vi "TempAcqSubVI.vi"(8 "error in (no error)":errorcluster, 11 "Data Cluster in":T1) -> (0 "error out":errorcluster, 2 "Temperature":dbl, 3 "Data Cluster out":T1)   [LabVIEW 2017]
uses:
  Controls/ShiftRegisterCluster.ctl
  <vilib>/DAQmx/read.llb/DAQmx Read (Analog DBL 1Chan 1Samp).vi
  <vilib>/DAQmx/miscellaneous.llb/DAQmx Fill In Error Info.vi
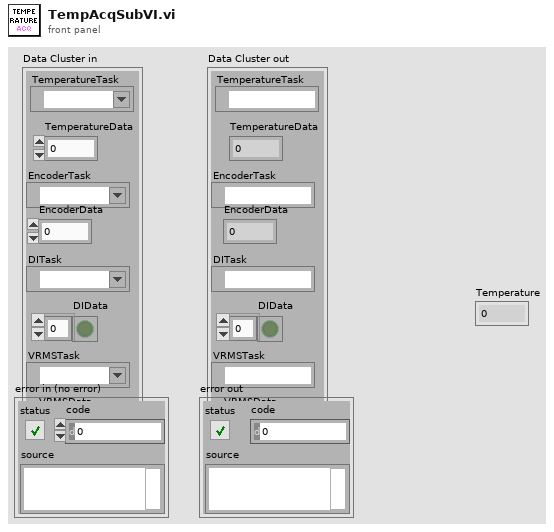
[diagram p1: front panel]
types:
  T1 = typedef "ShiftRegisterCluster.ctl" = cluster{"TemperatureTask":refnum<k21>, "TemperatureData":dbl, "EncoderTask":refnum<k21>, "EncoderData":dbl, "DITask":refnum<k21>, "DIData":bool[], "VRMSTask":refnum<k21>, "VRMSData":dbl, "FreqData":dbl}
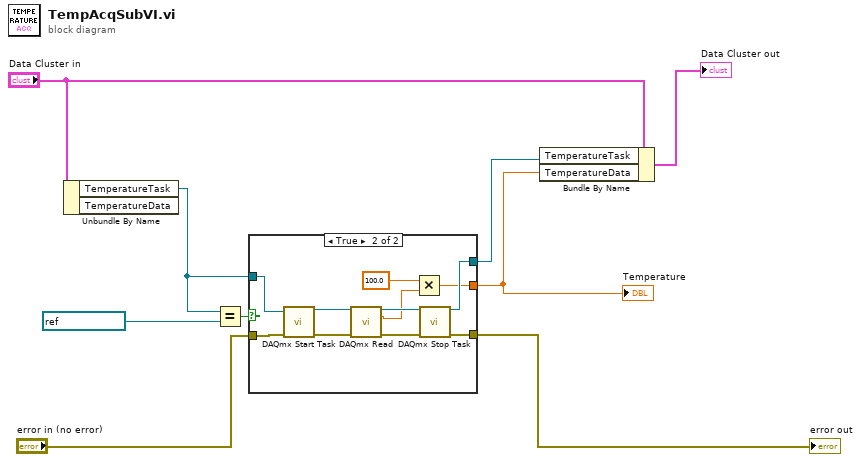
[diagram p0: block diagram]
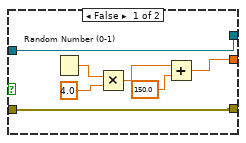
[diagram p2: hidden frame]
diagram:
  n1 = Unbundle By Name("Data Cluster in") -> ("TemperatureTask"=w3:refnum<k21>)  [unwired: 1 out]
  n2 = Equal?(x=w3, y=refnum<k21> "TempTask") -> (x = y?=w4:bool)
  n3 = case shown="True" w4 {
    tunnel: [w16 w27] -> w8
    tunnel: [w13 w26] -> w7
    tunnel: "error in (no error)" -> [w13 w25]
    tunnel: w3 -> [w16 w20]
    tunnel: [w10 w19] -> w2
    frame False {
      n4 = Random Number (0-1)() -> (number: 0 to 1=w15:dbl)
      n5 = Multiply(x=w15, y=4.0) -> (x*y=w12:dbl)
      n6 = Add(x=w12, y=150.0) -> (x+y=w10:dbl)
    }
    frame True {
      n7 = call <vilib>:"DAQmx Start Task.vi"("task/channels in"=w20, "error in"=w25) -> ("task out"=w24:refnum<k21>, "error out"=w23:errorcluster)  [unwired: 12 in]
      n8 = call-poly <vilib>:"DAQmx Read.vi"("task/channels in"=w24, "error in"=w23) -> ("task out"=w22:refnum<k21>, "data"=w18:dbl, "error out"=w21:errorcluster)  [unwired: 11 in]
      n9 = Multiply(x=100.0, y=w18) -> (x*y=w19:dbl)
      n10 = call <vilib>:"DAQmx Stop Task.vi"("task/channels in"=w22, "error in"=w21) -> ("task out"=w27:refnum<k21>, "error out"=w26:errorcluster)  [unwired: 12 in]
    }
  }
  "error out" <- w7
  "Temperature" <- w2
  n11 = Bundle By Name(cluster="Data Cluster in", "TemperatureTask"=w8, "TemperatureData"=w2) -> (→"Data Cluster out":T1)
